vi "numeric keypad (dbl).vi"(0 "Num Ref":refnum<vi>) -> ()   [LabVIEW 2014]
panel:
  in  "Show Value Initially":bool
  in  "Password":bool
  in  "Key +/-":bool
  in  "Divide":dbl=1.0
  in  "Key Reset":bool
  in  "Key .":bool
  in  "DOWN":bool
  in  "UP":bool
  in  "Number In":dbl
  in  "Cancel":bool
  in  "OK Button":bool
  out "Number":string
  in  "Key Clear":bool
  in  "Key DEL":bool
  in  "Key 0":bool
  in  "Key 9":bool
  in  "Key 8":bool
  in  "Key 7":bool
  in  "Key 6":bool
  in  "Key 5":bool
  in  "Key 4":bool
  in  "Key 3":bool
  in  "Key 2":bool
  in  "Key 1":bool
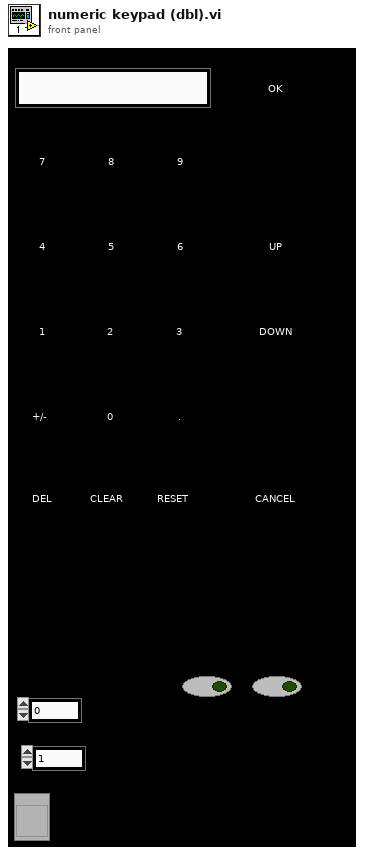
[diagram p1: front panel]
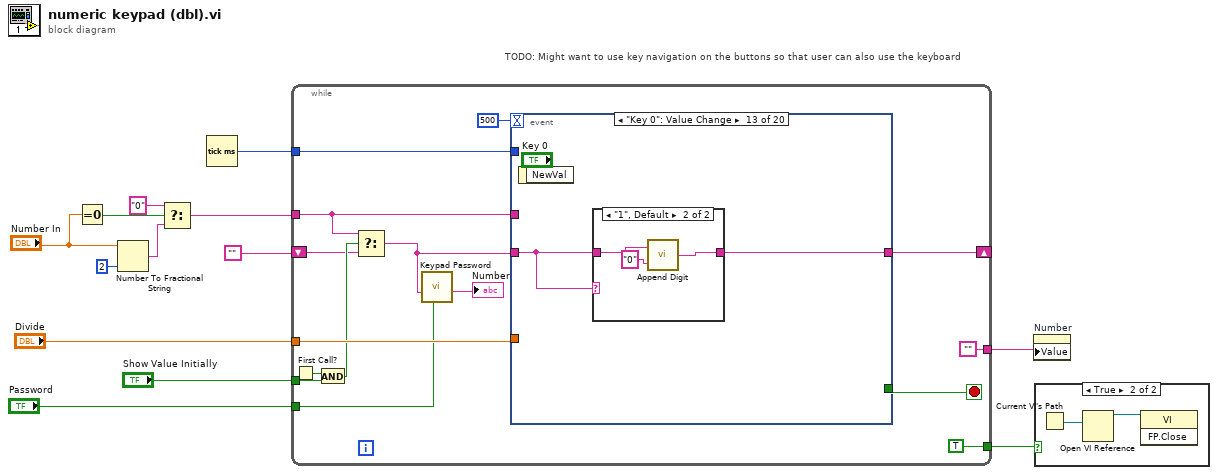
[diagram p0: block diagram]
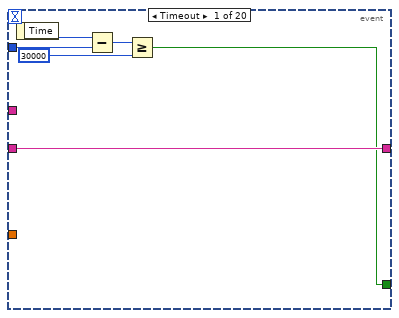
[diagram p3: hidden frame]
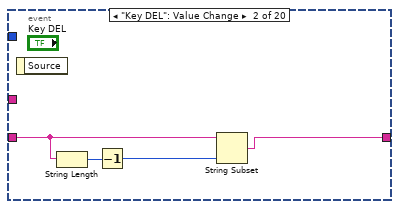
[diagram p4: hidden frame]
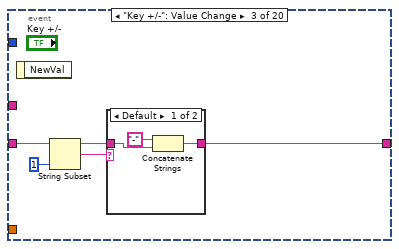
[diagram p5: hidden frame]
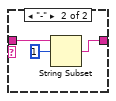
[diagram p6: hidden frame]
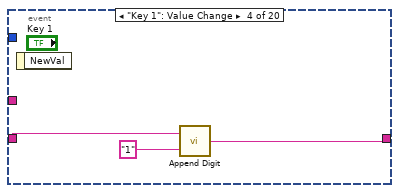
[diagram p7: hidden frame]
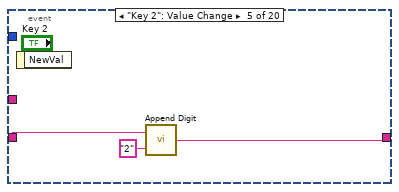
[diagram p8: hidden frame]
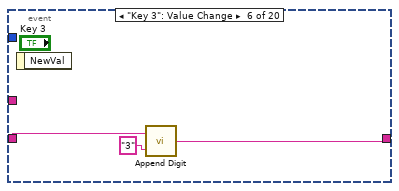
[diagram p9: hidden frame]
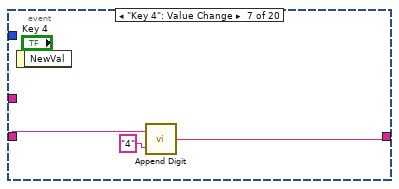
[diagram p10: hidden frame]
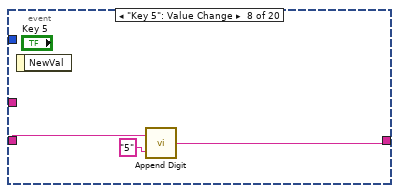
[diagram p11: hidden frame]
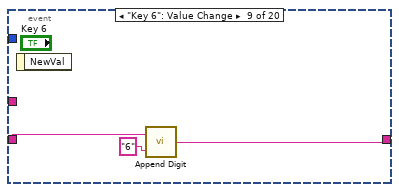
[diagram p12: hidden frame]
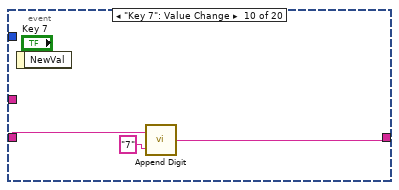
[diagram p13: hidden frame]
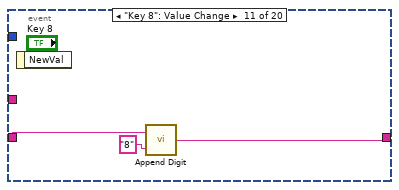
[diagram p14: hidden frame]
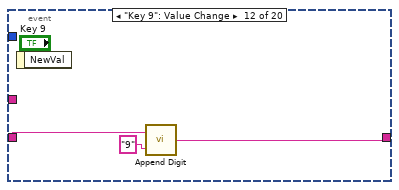
[diagram p15: hidden frame]
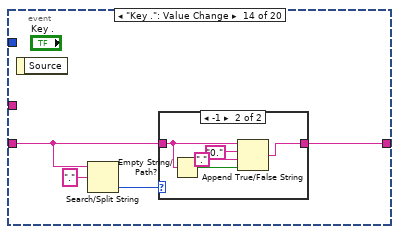
[diagram p17: hidden frame]
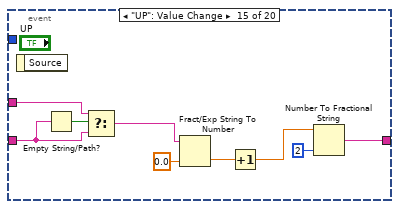
[diagram p19: hidden frame]
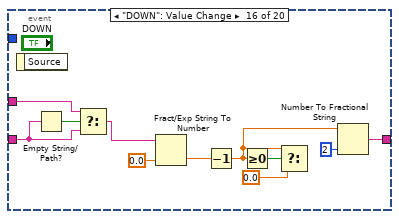
[diagram p20: hidden frame]
diagram:
  # "TODO: Might want to use key navigation on the buttons so that user can also use the keyboard"
  n1 = Equal To 0?(x="Number In") -> (x = 0?=w8:bool)
  n2 = Number To Fractional String(number="Number In", precision (6)=i16 2) -> (F-format string=w7:string)  [unwired: 2 in]
  n3 = Select(t="0", s=w8, f=w7) -> (s? t:f=w6:string)
  n4 = Tick Count (ms)() -> (millisecond timer value=w4:u32)
  n5 = while {
    shift-right: [w28] -> _
    shift-left: "" -> [w15]
    tunnel: [TRUE] -> w13
    tunnel: "Divide" -> [w25]
    tunnel: w6 -> [w21]
    tunnel: w4 -> [w23]
    tunnel: [""] -> w3
    tunnel: "Password" -> [w16]
    tunnel: "Show Value Initially" -> [w19]
    stop <- w27 stop-if-true
    n6 = First Call?() -> (First Call?: T/F=w18:bool)
    n7 = And(x=w18, y=w19) -> (x .and. y?=w20:bool)
    n8 = Select(t=w21, s=w20, f=w15) -> (s? t:f=w14:string)
    n9 = call "Keypad Password.vi"("Password?"=w16, "String In"=w14) -> ("String Out"=→"Number":string)  [unwired: 9 in]
    n10 = event shown="[12] \"Key 0\": Value Change" {
      selector: _ -> [_ _ _ _ _ _ _ _ _ _ _ _ _ _ _ _ _ _ _ _]
      dyn-events: _ -> [_ _ _ _ _ _ _ _ _ _ _ _ _ _ _ _ _ _ _ _]
      timeout: 500 -> [_ _ _ _ _ _ _ _ _ _ _ _ _ _ _ _ _ _ _ _]
      tunnel: w14 -> [w34 w37 w40 w51 w54 w57 w60 w63 w66 w69 w72 w75 w76 w83 w93 w104 _ _ w116 _]
      tunnel: [w34 w35 w39 w49 w52 w55 w58 w61 w64 w67 w70 w73 w77 w82 w97 w109 "" "" "" w125] -> w28
      tunnel: [w30 _ _ _ _ _ _ _ _ _ _ _ _ _ _ _ TRUE _ TRUE _] -> w27
      tunnel: w25 -> [_ _ _ _ _ _ _ _ _ _ _ _ _ _ _ _ _ _ w115 _]
      tunnel: w21 -> [_ _ _ _ _ _ _ _ _ _ _ _ _ _ w94 w102 _ _ _ w125]
      tunnel: w23 -> [w33 _ _ _ _ _ _ _ _ _ _ _ _ _ _ _ _ _ _ _]
      event Timeout {
        n11 = event-data() -> ("Time"=w29:u32)  [unwired: 1 in]
        n12 = Subtract(x=w29, y=w33) -> (x-y=w32:u32)
        n13 = Greater Or Equal?(x=w32, y=u32 30000) -> (x >= y?=w30:bool)
      }
      event "Key DEL": Value Change {
        n14 = event-data() -> ()  [unwired: 1 in, 1 out]
        n15 = String Length(string=w37) -> (length=w38:i32)
        n16 = Decrement(x=w38) -> (x-1=w36:i32)
        n17 = String Subset(string=w37, length (rest)=w36) -> (substring=w35:string)  [unwired: 1 in]
      }
      event "Key +/-": Value Change {
        n18 = event-data() -> ()  [unwired: 1 in, 1 out]
        n19 = String Subset(string=w40, length (rest)=1 ("length (rest)")) -> (substring=w41:string)  [unwired: 1 in]
        n20 = case shown="Default" w41 {
          tunnel: w40 -> [w43 w48]
          tunnel: [w45 w46] -> w39
          frame Default {
            n21 = Concatenate Strings("-" ("string"), w43) -> (w45:string)
          }
          frame "-" {
            n22 = String Subset(string=w48, offset (0)=1) -> (substring=w46:string)  [unwired: 1 in]
          }
        }
      }
      event "Key 1": Value Change {
        n23 = event-data() -> ()  [unwired: 1 in, 1 out]
        n24 = call "Append Digit.vi"("New Char"="1" ("string"), "Existing String"=w51) -> ("Resulting String"=w49:string)
      }
      event "Key 2": Value Change {
        n25 = event-data() -> ()  [unwired: 1 in, 1 out]
        n26 = call "Append Digit.vi"("New Char"="2" ("string"), "Existing String"=w54) -> ("Resulting String"=w52:string)
      }
      event "Key 3": Value Change {
        n27 = event-data() -> ()  [unwired: 1 in, 1 out]
        n28 = call "Append Digit.vi"("New Char"="3" ("string"), "Existing String"=w57) -> ("Resulting String"=w55:string)
      }
      event "Key 4": Value Change {
        n29 = event-data() -> ()  [unwired: 1 in, 1 out]
        n30 = call "Append Digit.vi"("New Char"="4" ("string"), "Existing String"=w60) -> ("Resulting String"=w58:string)
      }
      event "Key 5": Value Change {
        n31 = event-data() -> ()  [unwired: 1 in, 1 out]
        n32 = call "Append Digit.vi"("New Char"="5" ("string"), "Existing String"=w63) -> ("Resulting String"=w61:string)
      }
      event "Key 6": Value Change {
        n33 = event-data() -> ()  [unwired: 1 in, 1 out]
        n34 = call "Append Digit.vi"("New Char"="6" ("string"), "Existing String"=w66) -> ("Resulting String"=w64:string)
      }
      event "Key 7": Value Change {
        n35 = event-data() -> ()  [unwired: 1 in, 1 out]
        n36 = call "Append Digit.vi"("New Char"="7" ("string"), "Existing String"=w69) -> ("Resulting String"=w67:string)
      }
      event "Key 8": Value Change {
        n37 = event-data() -> ()  [unwired: 1 in, 1 out]
        n38 = call "Append Digit.vi"("New Char"="8" ("string"), "Existing String"=w72) -> ("Resulting String"=w70:string)
      }
      event "Key 9": Value Change {
        n39 = event-data() -> ()  [unwired: 1 in, 1 out]
        n40 = call "Append Digit.vi"("New Char"="9" ("string"), "Existing String"=w75) -> ("Resulting String"=w73:string)
      }
      event "Key 0": Value Change {
        n41 = event-data() -> ()  [unwired: 1 in, 1 out]
        n42 = case shown="\"1\", Default" w76 {
          tunnel: w76 -> [w78 w81]
          tunnel: [w78 w79] -> w77
          frame "0" {
          }
          frame "1", Default {
            n43 = call "Append Digit.vi"("New Char"="0" ("string"), "Existing String"=w81) -> ("Resulting String"=w79:string)
          }
        }
      }
      event "Key .": Value Change {
        n44 = event-data() -> ()  [unwired: 1 in, 1 out]
        n45 = Search/Split String(string=w83, search string/char (-)=".") -> (offset of match=w84:i32)  [unwired: 1 in, 2 out]
        n46 = case shown="-1" w84 {
          tunnel: w83 -> [w86 w91]
          tunnel: [w86 w90] -> w82
          frame 0, Default {
          }
          frame -1 {
            n47 = Empty String/Path?(string/path=w91) -> (empty?=w87:bool)
            n48 = Append True/False String(1:w87, 2:"." ("string"), 3:"0." ("string"), 4:w91) -> (0:w90:string)
          }
        }
      }
      event "UP": Value Change {
        n49 = event-data() -> ()  [unwired: 1 in, 1 out]
        n50 = Empty String/Path?(string/path=w93) -> (empty?=w95:bool)
        n51 = Select(t=w94, s=w95, f=w93) -> (s? t:f=w92:string)
        n52 = Fract/Exp String To Number(string=w92, default (0 dbl)=0.0 ("default (0 I32)")) -> (number=w99:dbl)  [unwired: 2 in, 1 out]
        n53 = Increment(x=w99) -> (x+1=w98:dbl)
        n54 = Number To Fractional String(number=w98, precision (6)=i16 2) -> (F-format string=w97:string)  [unwired: 2 in]
      }
      event "DOWN": Value Change {
        n55 = event-data() -> ()  [unwired: 1 in, 1 out]
        n56 = Empty String/Path?(string/path=w104) -> (empty?=w105:bool)
        n57 = Select(t=w102, s=w105, f=w104) -> (s? t:f=w103:string)
        n58 = Fract/Exp String To Number(string=w103, default (0 dbl)=0.0 ("default (0 I32)")) -> (number=w110:dbl)  [unwired: 2 in, 1 out]
        n59 = Decrement(x=w110) -> (x-1=w101:dbl)
        n60 = Greater Or Equal To 0?(x=w101) -> (x >= 0?=w108:bool)
        n61 = Select(t=w101, s=w108, f=0.0) -> ()  [unwired: 1 out]
        n62 = Number To Fractional String(number=w101, precision (6)=i16 2) -> (F-format string=w109:string)  [unwired: 2 in]
      }
      event "Cancel": Value Change {
        n63 = event-data() -> ()  [unwired: 1 in, 6 out]
      }
      event "Key Clear": Value Change {
        n64 = event-data() -> ()  [unwired: 1 in, 6 out]
      }
      event "OK Button": Value Change {
        n65 = event-data() -> ()  [unwired: 1 in, 1 out]
        n66 = case shown="\"0\", Default" w116 {
          selector: w116 -> [_ w123]
          tunnel: w115 -> [_ w124]
          frame "" {
          }
          frame "0", Default {
            n67 = Fract/Exp String To Number(string=w123, default (0 dbl)=0.0 ("default (0 DBL)")) -> (number=w121:dbl)  [unwired: 2 in, 1 out]
            n68 = Multiply(x=w121, y=w124) -> (x*y=w119:dbl)
            n69 = property class="Num"(reference="Num Ref", "Value (Signaling)"=w119) -> ()  [unwired: 1 in, 2 out]
          }
        }
      }
      event "Key Reset": Value Change {
        n70 = event-data() -> ()  [unwired: 1 in, 1 out]
      }
    }
  }
  n71 = property on="Number" class="Str"("Value"=w3) -> ()  [unwired: 2 in, 2 out]
  n72 = case shown="True" w13 {
    frame False {
    }
    frame True {
      n73 = Current VI's Path() -> (path=w127:path)
      n74 = Open VI Reference(vi path=w127) -> (vi reference=w126:refnum<vi>)  [unwired: 5 in, 1 out]
      n75 = invoke class="VI" method="FP.Close"(reference=w126) -> ()  [unwired: 2 in, 3 out]
    }
  }
